vi "Add Member to Database.vi"(8 "error in (no error)":errorcluster, 10 "UI data":variant, 11 "PluginWithDatabase in":refnum<class "PluginWithDatabase.lvclass">) -> (0 "error out":errorcluster, 3 "PluginWithDatabase out":refnum<class "PluginWithDatabase.lvclass">)   [LabVIEW 2015, in "ActorManagement.lvlib" / "PluginWithDatabase.lvclass"]
uses:
  PluginWithDatabase/PluginWithDatabase.lvclass
  Plugin.lvclass/Plugin.ctl
  PluginWithDatabase/PluginWithDatabase.lvclass/PluginWithDatabase.ctl
  DatabaseManagement/Database.lvclass
  UserManagement/Model/Model.lvclass
  Plugin.lvclass
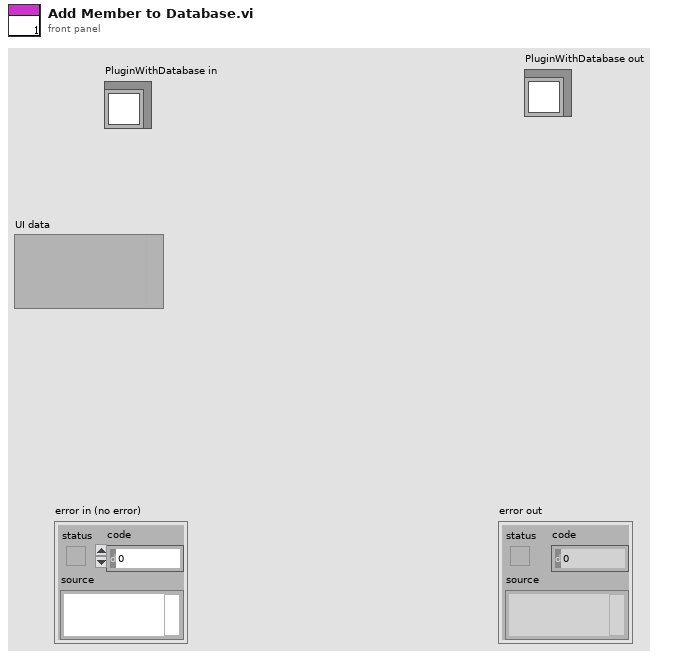
[diagram p1: front panel]
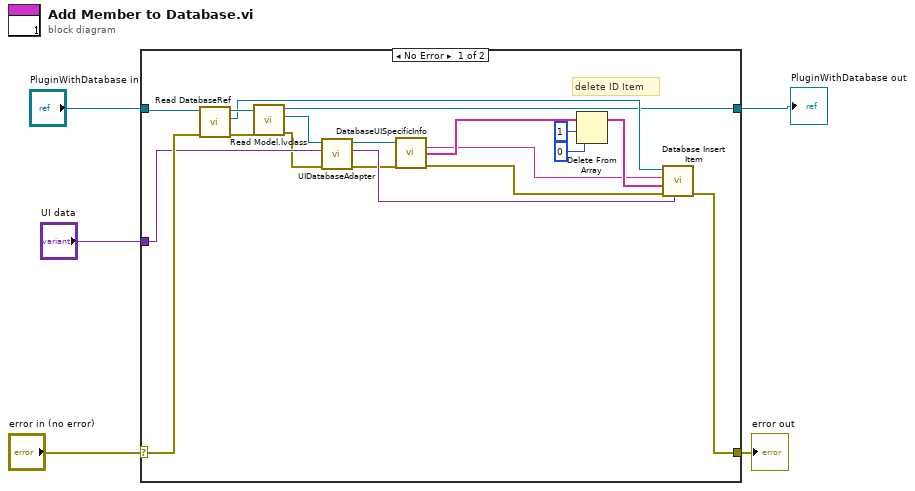
[diagram p0: block diagram]
diagram:
  n1 = case shown="No Error" "error in (no error)" {
    selector: "error in (no error)" -> [w19 w26]
    tunnel: [w24 w26] -> w4
    tunnel: [w6 w25] -> w1
    tunnel: "PluginWithDatabase in" -> [w20 w25]
    tunnel: "UI data" -> [w15 _]
    frame No Error {
      # "delete ID Item"
      n2 = call "Read DatabaseRef.vi"("error in (no error)"=w19, "Plugin in"=w20) -> ("error out"=w17:errorcluster, "Database.lvlib:Database"=w9:refnum<class "Database.lvclass">, "Plugin out"=w18:refnum<class "PluginWithDatabase.lvclass">)  [unwired: 7 in]
      n3 = call "Read Model.lvclass.vi"("error in (no error)"=w17, "PluginWithDatabase in"=w18) -> ("error out"=w14:errorcluster, "UserManagement.lvlib:Model"=w16:refnum<class "Model.lvclass">, "PluginWithDatabase out"=w6:refnum<class "PluginWithDatabase.lvclass">)  [unwired: 7 in]
      n4 = call-dynamic "UIDatabaseAdapter.vi"("error in (no error)"=w14, "UI Data"=w15, "Model.lvclass"=w16) -> ("error out"=w11:errorcluster, "Database Data"=w13:variant, "Model.lvclass out"=w12:refnum<class "Model.lvclass">)  [unwired: 6 in]
      n5 = call-dynamic "DatabaseUISpecificInfo.vi"("Model.lvclass"=w12, "error in (no error)"=w11) -> ("TableName"=w8:string, "TableItems"=w10:string[], "error out"=w7:errorcluster)  [unwired: 9 in, 2 out]
      n6 = Delete From Array(array=w10, length=1, index=0) -> (array with subset deleted=w21:string[])  [unwired: 1 out]
      n7 = call "Database Insert Item.vi"("data"=w13, "error in (no error)"=w7, "columns"=w21, "table"=w8, "object in"=w9) -> ("error out"=w24:errorcluster)  [unwired: 5 in, 1 out]
    }
    frame Error {
    }
  }
  "error out" <- w4
  "PluginWithDatabase out" <- w1
